vi "DSF.Engine.Memory.Cache.Transfer.Get Largest Count.All Types.vi"(8 "error in (no error)":errorcluster, 10 "Data Type Counts in":T1 {"U64" format="%d elements"; "U32" format="%d elements"; "U16" format="%d elements"; "U8" format="%d elements"; "I64" format="%d elements"; "I32" format="%d elements"; "I16" format="%d elements"; "I8" format="%d elements"; "DBL" format="%d elements"; "SGL" format="%d elements"; "Bool" format="%d elements"}, 11 "Transfer Cache in":refnum<class "DSF.Engine.Memory.Cache.Transfer.lvclass">) -> (0 "error out":errorcluster, 2 "Data Type Counts out":T1 {"U64" format="%d elements"; "U32" format="%d elements"; "U16" format="%d elements"; "U8" format="%d elements"; "I64" format="%d elements"; "I32" format="%d elements"; "I16" format="%d elements"; "I8" format="%d elements"; "DBL" format="%d elements"; "SGL" format="%d elements"; "Bool" format="%d elements"}, 3 "Transfer Cache out":refnum<class "DSF.Engine.Memory.Cache.Transfer.lvclass">)   [LabVIEW 2016, in "DSF.Engine.lvlib" / "DSF.Engine.Memory.Cache.Transfer.lvclass"]
uses:
  DSF.Engine.Memory.Cache.Transfer.lvclass
  Typedefs/DSF.Shared.Data Type Counts.ctl
  DSF.Engine.Memory.Cache.Transfer.lvclass/DSF.Engine.Memory.Cache.Transfer.ctl
  DSF.Shared.lvlib
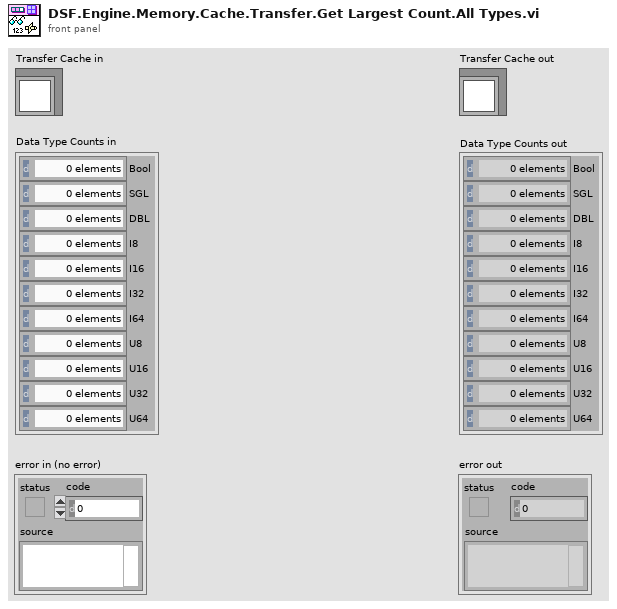
[diagram p1: front panel]
types:
  T1 = typedef "DSF.Shared.lvlib/DSF.Shared.Data Type Counts.ctl" = cluster{"Bool":u64, "SGL":u64, "DBL":u64, "I8":u64, "I16":u64, "I32":u64, "I64":u64, "U8":u64, "U16":u64, "U32":u64, "U64":u64}
  T2 = typedef "DSF.Engine.lvlib/DSF.Engine.Buffer Channel Configuration.ctl" = cluster{"data type":T3, "offset":u64, "count":u64, "index":u64}
  T3 = typedef "DSF.Shared.lvlib/DSF.Shared.Data Type.ctl" = enum8{"Bool", "SGL", "DBL", "I8", "I16", "I32", "I64", "U8", "U16", "U32", "U64"}
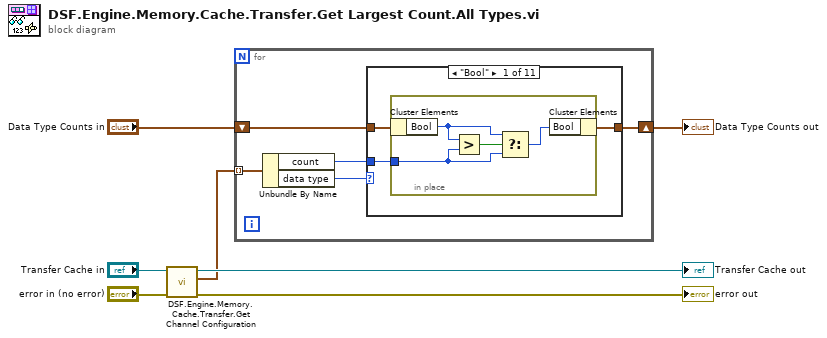
[diagram p0: block diagram]
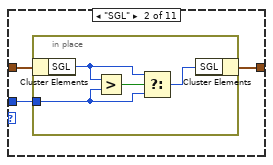
[diagram p2: hidden frame]
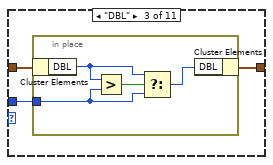
[diagram p3: hidden frame]
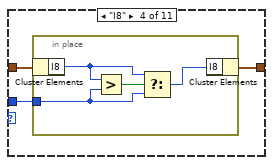
[diagram p4: hidden frame]
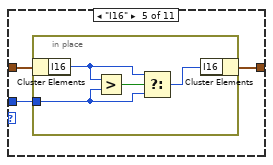
[diagram p5: hidden frame]
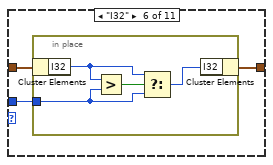
[diagram p6: hidden frame]
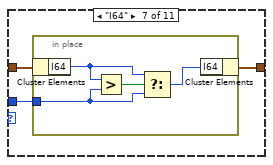
[diagram p7: hidden frame]
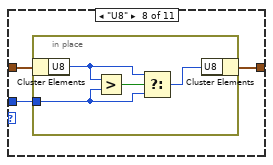
[diagram p8: hidden frame]
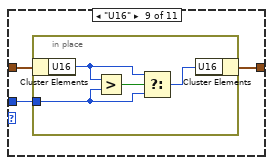
[diagram p9: hidden frame]
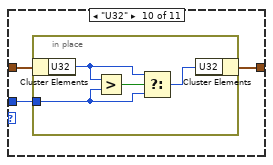
[diagram p10: hidden frame]
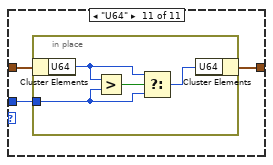
[diagram p11: hidden frame]
diagram:
  n1 = call "DSF.Engine.Memory.Cache.Transfer.Get Channel Configuration.vi"("error in (no error)"="error in (no error)", "Transfer Cache in"="Transfer Cache in") -> ("error out"=→"error out":errorcluster, "Channel Configuration"=w3:T2[], "Transfer Cache out"=→"Transfer Cache out":refnum<class "DSF.Engine.Memory.Cache.Transfer.lvclass">)  [unwired: 7 in]
  n2 = for {
    tunnel: w3 -> [w12] mode=indexing
    shift-right: [w8] -> w1
    shift-left: "Data Type Counts in" -> [w10]
    n3 = Unbundle By Name(w12) -> ("count"=w9:u64, "data type"=w11:T3)
    n4 = case shown="\"Bool\"" w11 {
      tunnel: w10 -> [w15 w22 w29 w36 w43 w50 w57 w64 w71 w78 w85]
      tunnel: w9 -> [w14 w21 w28 w35 w42 w49 w56 w63 w70 w77 w84]
      tunnel: [w13 w20 w27 w34 w41 w48 w55 w62 w69 w76 w83] -> w8
      frame "Bool" {
        n5 = in-place {
          in-place-border: w14 -> [w17]
          n6 = in-place-cluster #1(w15) -> ("Bool"=w18:u64)
          n7 = Greater?(x=w18, y=w17) -> (0:w19:bool)
          n8 = Select(t=w18, s=w19, f=w17) -> (s? t:f=w16:u64)
          n9 = in-place-cluster #1("Bool"=w16) -> (w13:T1)
        }
      }
      frame "SGL" {
        n10 = in-place {
          in-place-border: w21 -> [w24]
          n11 = in-place-cluster #2(w22) -> ("SGL"=w25:u64)
          n12 = Greater?(x=w25, y=w24) -> (0:w26:bool)
          n13 = Select(t=w25, s=w26, f=w24) -> (s? t:f=w23:u64)
          n14 = in-place-cluster #2("SGL"=w23) -> (w20:T1)
        }
      }
      frame "DBL" {
        n15 = in-place {
          in-place-border: w28 -> [w31]
          n16 = in-place-cluster #3(w29) -> ("DBL"=w32:u64)
          n17 = Greater?(x=w32, y=w31) -> (0:w33:bool)
          n18 = Select(t=w32, s=w33, f=w31) -> (s? t:f=w30:u64)
          n19 = in-place-cluster #3("DBL"=w30) -> (w27:T1)
        }
      }
      frame "I8" {
        n20 = in-place {
          in-place-border: w35 -> [w38]
          n21 = in-place-cluster #4(w36) -> ("I8"=w39:u64)
          n22 = Greater?(x=w39, y=w38) -> (0:w40:bool)
          n23 = Select(t=w39, s=w40, f=w38) -> (s? t:f=w37:u64)
          n24 = in-place-cluster #4("I8"=w37) -> (w34:T1)
        }
      }
      frame "I16" {
        n25 = in-place {
          in-place-border: w42 -> [w45]
          n26 = in-place-cluster #5(w43) -> ("I16"=w46:u64)
          n27 = Greater?(x=w46, y=w45) -> (0:w47:bool)
          n28 = Select(t=w46, s=w47, f=w45) -> (s? t:f=w44:u64)
          n29 = in-place-cluster #5("I16"=w44) -> (w41:T1)
        }
      }
      frame "I32" {
        n30 = in-place {
          in-place-border: w49 -> [w52]
          n31 = in-place-cluster #6(w50) -> ("I32"=w53:u64)
          n32 = Greater?(x=w53, y=w52) -> (0:w54:bool)
          n33 = Select(t=w53, s=w54, f=w52) -> (s? t:f=w51:u64)
          n34 = in-place-cluster #6("I32"=w51) -> (w48:T1)
        }
      }
      frame "I64" {
        n35 = in-place {
          in-place-border: w56 -> [w59]
          n36 = in-place-cluster #7(w57) -> ("I64"=w60:u64)
          n37 = Greater?(x=w60, y=w59) -> (0:w61:bool)
          n38 = Select(t=w60, s=w61, f=w59) -> (s? t:f=w58:u64)
          n39 = in-place-cluster #7("I64"=w58) -> (w55:T1)
        }
      }
      frame "U8" {
        n40 = in-place {
          in-place-border: w63 -> [w66]
          n41 = in-place-cluster #8(w64) -> ("U8"=w67:u64)
          n42 = Greater?(x=w67, y=w66) -> (0:w68:bool)
          n43 = Select(t=w67, s=w68, f=w66) -> (s? t:f=w65:u64)
          n44 = in-place-cluster #8("U8"=w65) -> (w62:T1)
        }
      }
      frame "U16" {
        n45 = in-place {
          in-place-border: w70 -> [w73]
          n46 = in-place-cluster #9(w71) -> ("U16"=w74:u64)
          n47 = Greater?(x=w74, y=w73) -> (0:w75:bool)
          n48 = Select(t=w74, s=w75, f=w73) -> (s? t:f=w72:u64)
          n49 = in-place-cluster #9("U16"=w72) -> (w69:T1)
        }
      }
      frame "U32" {
        n50 = in-place {
          in-place-border: w77 -> [w80]
          n51 = in-place-cluster #10(w78) -> ("U32"=w81:u64)
          n52 = Greater?(x=w81, y=w80) -> (0:w82:bool)
          n53 = Select(t=w81, s=w82, f=w80) -> (s? t:f=w79:u64)
          n54 = in-place-cluster #10("U32"=w79) -> (w76:T1)
        }
      }
      frame "U64" {
        n55 = in-place {
          in-place-border: w84 -> [w87]
          n56 = in-place-cluster #11(w85) -> ("U64"=w88:u64)
          n57 = Greater?(x=w88, y=w87) -> (0:w89:bool)
          n58 = Select(t=w88, s=w89, f=w87) -> (s? t:f=w86:u64)
          n59 = in-place-cluster #11("U64"=w86) -> (w83:T1)
        }
      }
    }
  }
  "Data Type Counts out" <- w1
